vi "Remove_Char_at_ends.vi"(1 "String in":string, 2 "Characters to remove":string="_") -> (0 "String out":string)   [LabVIEW 2010]
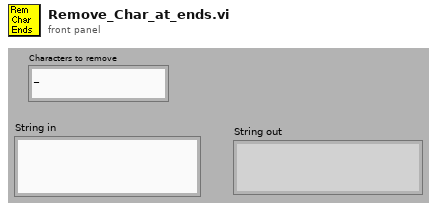
[diagram p1: front panel]
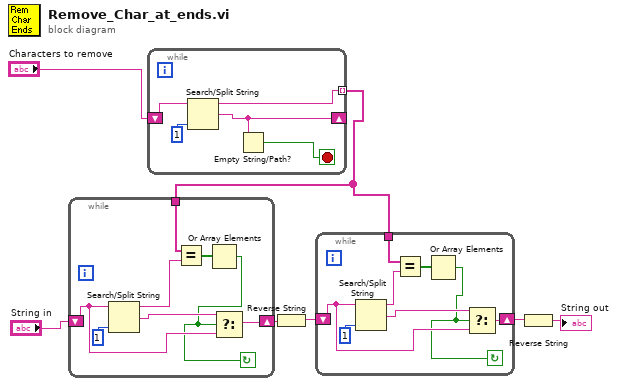
[diagram p0: block diagram]
diagram:
  n1 = while {
    shift-left: "Characters to remove" -> [w11]
    shift-right: [w9] -> _
    tunnel: [w8] -> w1 mode=indexing
    stop <- w10 stop-if-true
    n2 = Search/Split String(string=w11, offset (0)=1 ("length")) -> (substring before match=w8:string, match + rest of string=w9:string)  [unwired: 2 out]
    n3 = Empty String/Path?(string/path=w9) -> (empty?=w10:bool)
  }
  n4 = while {
    shift-left: "String in" -> [w18]
    shift-right: [w17] -> w3
    tunnel: w1 -> [w15]
    stop <- w13 continue-if-true
    n5 = Search/Split String(string=w18, offset (0)=1 ("length")) -> (substring before match=w16:string, match + rest of string=w19:string)  [unwired: 2 out]
    n6 = Equal?(x=w15, y=w16) -> (x = y?=w14:bool[])
    n7 = Or Array Elements(Boolean array=w14) -> (logical OR=w13:bool)
    n8 = Select(t=w19, s=w13, f=w18) -> (s? t:f=w17:string)
  }
  n9 = Reverse String(1:w3) -> (0:w4:string)
  n10 = while {
    shift-left: w4 -> [w26]
    shift-right: [w25] -> w5
    tunnel: w1 -> [w22]
    stop <- w21 continue-if-true
    n11 = Search/Split String(string=w26, offset (0)=1 ("length")) -> (substring before match=w23:string, match + rest of string=w27:string)  [unwired: 2 out]
    n12 = Equal?(x=w22, y=w23) -> (x = y?=w24:bool[])
    n13 = Or Array Elements(Boolean array=w24) -> (logical OR=w21:bool)
    n14 = Select(t=w27, s=w21, f=w26) -> (s? t:f=w25:string)
  }
  n15 = Reverse String(1:w5) -> (0:→"String out":string)
